vi "OutOfRangeColor.vi"(11 "Array":refnum<vi>[](array[refnum])) -> ()   [LabVIEW 2018, in "Testing UI 2.lvlib"]
uses:
  Testing UI 2.lvlib
  feecbcb5-ab4f-447a-b243-a0081445e8de.vi
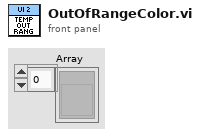
[diagram p1: front panel]
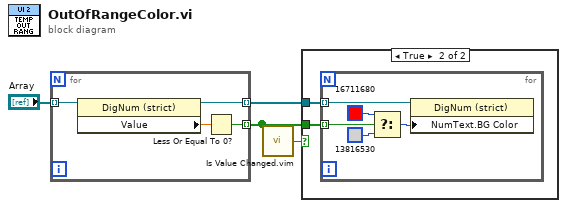
[diagram p0: block diagram]
diagram:
  n1 = for {
    tunnel: "Array" -> [w7] mode=indexing
    tunnel: [w6] -> w3 mode=indexing
    tunnel: [w5] -> w4 mode=indexing
    n2 = property class="DigNum (strict)"(reference=w7) -> (reference out=w5:refnum<vi>, "Value"=w8:dbl)  [unwired: 1 in, 1 out]
    n3 = Less Or Equal To 0?(x=w8) -> (x <= 0?=w6:bool)
  }
  n4 = call "Is Value Changed.vim"("value"=w3) -> ("changed or first call?"=w2:bool)
  n5 = case shown="True" w2 {
    tunnel: w3 -> [_ w10]
    tunnel: w4 -> [_ w9]
    frame False {
    }
    frame True {
      n6 = for {
        tunnel: w10 -> [w13] mode=indexing
        tunnel: w9 -> [w11] mode=indexing
        n7 = Select(t=u32 16711680, s=w13, f=u32 13816530) -> (s? t:f=w12:u32)
        n8 = property class="DigNum (strict)"(reference=w11, "NumText.BG Color"=w12) -> ()  [unwired: 1 in, 2 out]
      }
    }
  }
